vi "Beta 2.0.vi"() -> ()   [LabVIEW 2011]
panel:
  in  "Stop":bool
  in  "Browse":bool
  out "XY Graph":cluster{dbl[], dbl[]}(graph)
  out "Original Image":T1(plugin-control)
  out "Path to Image":path
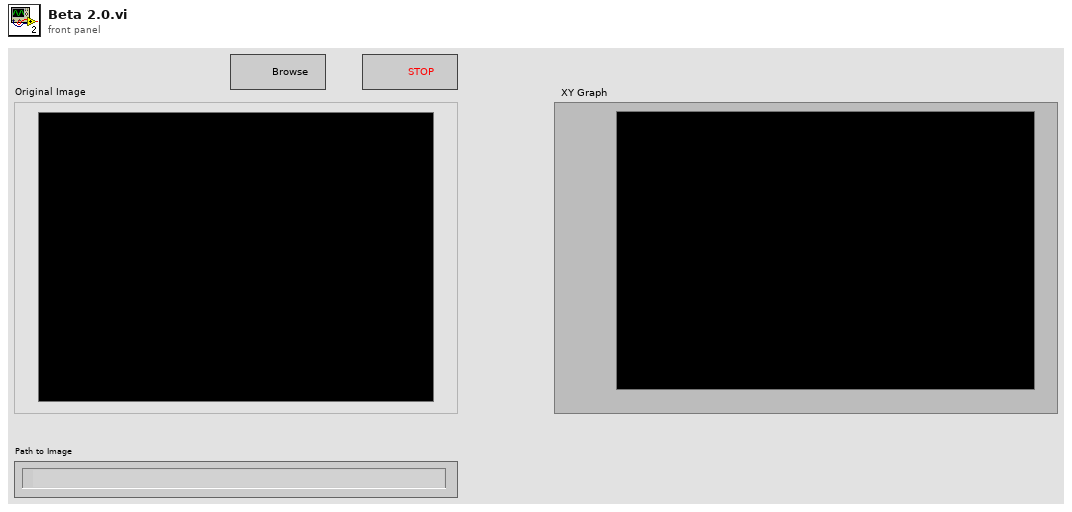
[diagram p1: front panel]
types:
  T1 = typedef "IMAQ Image.ctl" = refnum<image>
  T2 = typedef "Image Type" = u32
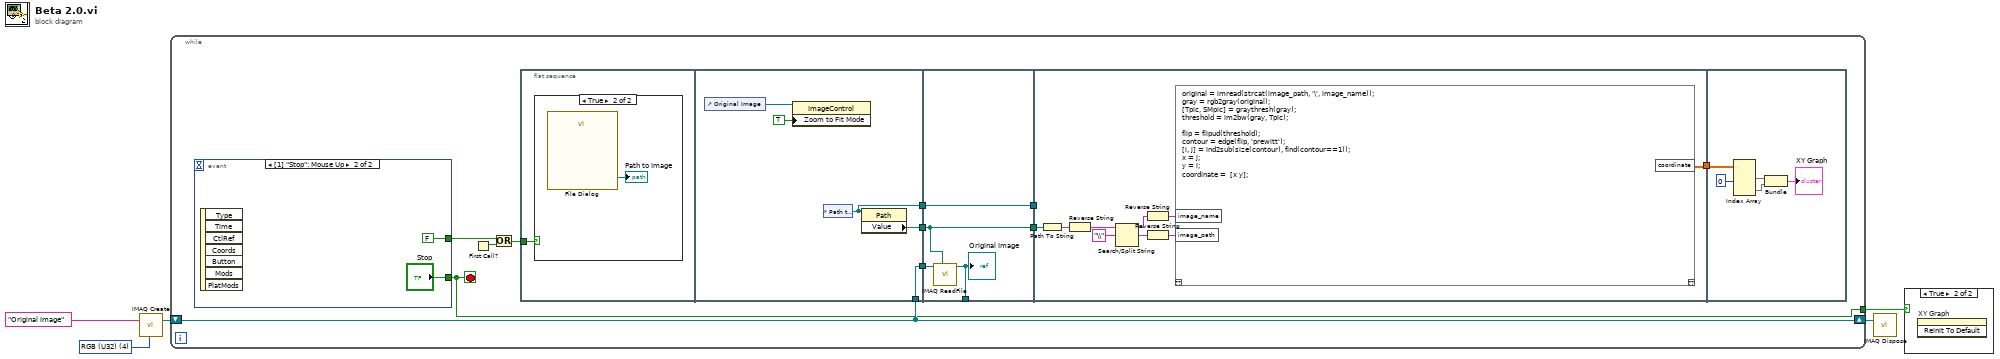
[diagram p0: block diagram]
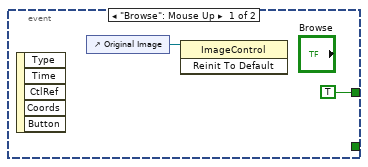
[diagram p3: hidden frame]
diagram:
  w4 = T2 4 items=["Grayscale (U8)", "Grayscale (I16)", "Grayscale (SGL)", "Complex (CSG)", "RGB (U32)", "HSL (U32)", "RGB (U64)", "Grayscale (U16)"] ("Image Type")
  n1 = call "IMAQ Create"("Image Name"="Original Image", "Image Type"=w4) -> ("New Image"=w3:T1)  [unwired: 3 in, 1 out]
  n2 = while {
    shift-right: [w7] -> w2
    shift-left: w3 -> [w7]
    tunnel: [w6] -> w1
    stop <- w6 stop-if-true
    n3 = event shown="[1] \"Stop\": Mouse Up" {
      selector: _ -> [_ _]
      dyn-events: _ -> [_ _]
      timeout: _ -> [_ _]
      tunnel: [TRUE FALSE] -> w13
      tunnel: [_ "Stop"] -> w6
      event "Browse": Mouse Up {
        n4 = event-data() -> ()  [unwired: 1 in, 5 out]
        n5 = control-ref of="Original Image"() -> (w18:refnum<vi>)
        n6 = invoke class="ImageControl" method="Reinit To Default"(reference=w18) -> ()  [unwired: 2 in, 3 out]
      }
      event "Stop": Mouse Up {
        n7 = event-data() -> ()  [unwired: 1 in, 7 out]
      }
    }
    n8 = First Call?() -> (First Call?: T/F=w11:bool)
    n9 = Or(x=w13, y=w11) -> (x .or. y?=w10:bool)
    n10 = flat-sequence {
      tunnel: w10 -> [w21]
      tunnel: [w23] -> w14
      tunnel: [w25] -> w12
      tunnel: [w24] -> w9
      tunnel: w7 -> [w23]
      tunnel: [w29] -> w16
      tunnel: [w31] -> _
      tunnel: w14 -> [w30]
      tunnel: w12 -> [w29]
      tunnel: w9 -> [w28]
      tunnel: [w28] -> w8
      tunnel: w16 -> [_]
      tunnel: [w33] -> w15
      tunnel: w8 -> [w32]
      tunnel: w15 -> [w45]
      frame #0 {
        n11 = case shown="True" w21 {
          frame False {
          }
          frame True {
            n12 = call "File Dialog"() -> ("selected path"=→"Path to Image":path)  [unwired: 12 in, 3 out]
          }
        }
      }
      frame #1 {
        n13 = control-ref of="Original Image"() -> (w27:refnum<vi>)
        n14 = property class="ImageControl"(reference=w27, "Zoom to Fit Mode"=TRUE) -> ()  [unwired: 1 in, 2 out]
        n15 = control-ref of="Path to Image"() -> (w25:refnum<vi>)
        n16 = property class="Path"(reference=w25) -> ("Value"=w24:path)  [unwired: 1 in, 2 out]
      }
      frame #2 {
        n17 = call "IMAQ ReadFile"("File Path"=w28, "Image"=w30) -> ("Image Out"=w31:T1)  [unwired: 5 in, 4 out]
        "Original Image" <- w31
      }
      frame #3 {
        n18 = Path To String(path=w32) -> (string=w40:string)
        n19 = Reverse String(1:w40) -> (0:w39:string)
        n20 = Search/Split String(string=w39, search string/char (-)="\\") -> (substring before match=w37:string, match + rest of string=w36:string)  [unwired: 1 in, 1 out]
        n21 = Reverse String(1:w37) -> (0:w35:string)
        n22 = Reverse String(1:w36) -> (0:w34:string)
        n23 = script code="original = imread(strcat(image_path, '\\', image_name));\ngray = rgb2gray(original);\n[Tpic, SMpic] = graythresh(gray);\nthreshold = im2bw(gray, Tpic);\n\nflip = flipud(threshold);\ncontour = edge(flip, 'prewitt');\n[i, j] = ind2sub(size(contour), find(contour==1));\nx = j;\ny = i;\ncoordinate =  [x y];"("image_name"=w35, "image_path"=w34) -> ("coordinate"=w33:dbl[][])  [unwired: 1 in, 1 out]
      }
      frame #4 {
        n24 = Index Array(array=w45, index (col) #1=0 ("disabled index (col)")) -> (element #1=w43:dbl[], element #2=w42:dbl[])  [unwired: 3 in]
        n25 = Bundle(w43, w42) -> (→"XY Graph":cluster{dbl[], dbl[]})  [unwired: 1 in]
      }
    }
  }
  n26 = call "IMAQ Dispose"("Image"=w2) -> ()  [unwired: 5 in, 1 out]
  n27 = case shown="True" w1 {
    frame False {
    }
    frame True {
      n28 = invoke on="XY Graph" class="XYGraph (strict)" method="Reinit To Default"() -> ()  [unwired: 3 in, 3 out]
    }
  }
